vi "configureTriggering.vi"(8 "error in (no error)":errorcluster, 10 "channel":i32, 11 "K2602 in":refnum<class "K2602.lvclass">) -> (0 "error out":errorcluster, 3 "K2602 out":refnum<class "K2602.lvclass">)   [LabVIEW 2009, in "Hardware.lvlib" / "Channels.lvlib" / "K2602.lvclass"]
uses:
  K2602.lvclass
  K2602.lvclass/K2602.ctl
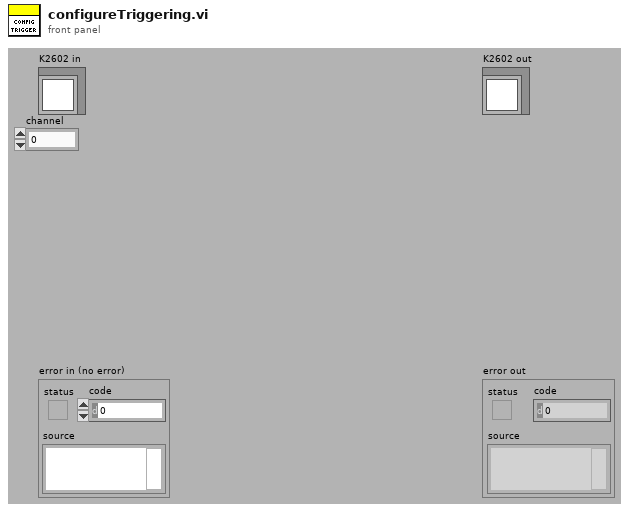
[diagram p1: front panel]
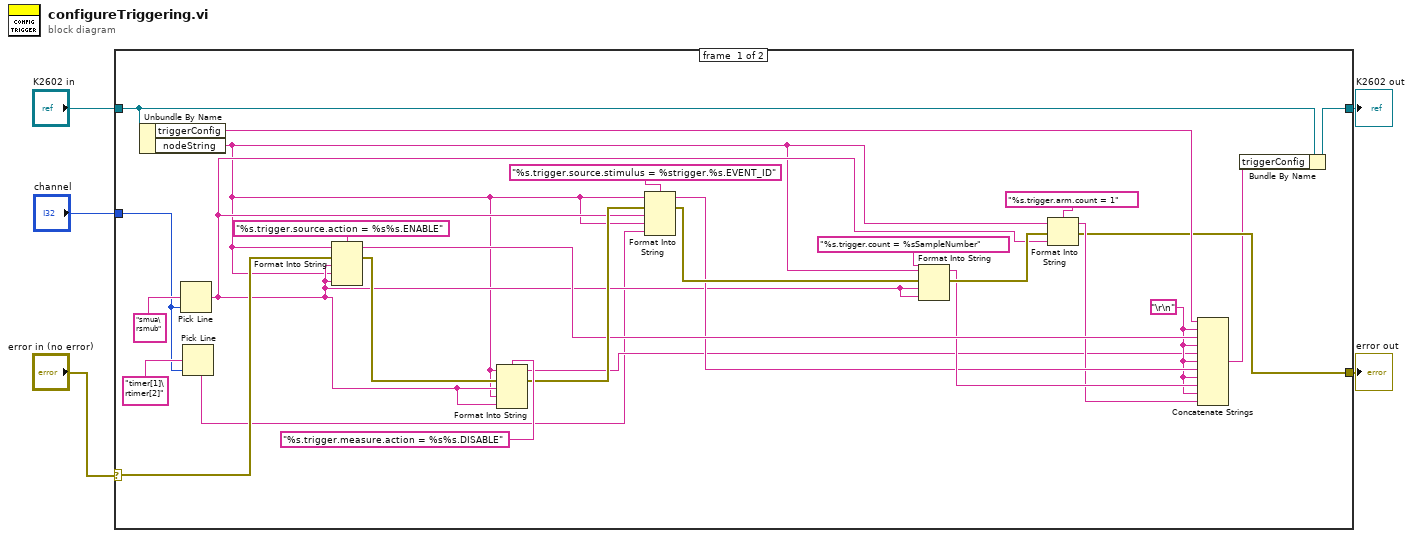
[diagram p0: block diagram]
diagram:
  n1 = case shown="No Error" "error in (no error)" {
    selector: "error in (no error)" -> [w30 w34]
    tunnel: [w14 w34] -> w4
    tunnel: [w11 w33] -> w2
    tunnel: "K2602 in" -> [w12 w33]
    tunnel: "channel" -> [w24 _]
    frame #0 {
      w10 = "\r\n"
      n2 = Unbundle By Name(w12) -> ("triggerConfig"=w19:string, "nodeString"=w6:string)
      n3 = Pick Line(multi-line string="smua\rsmub" ("options"), line index=w24) -> (output string=w8:string)  [unwired: 1 out]
      n4 = Pick Line(multi-line string="timer[1]\rtimer[2]" ("options"), line index=w24) -> (output string=w7:string)  [unwired: 1 out]
      n5 = Format Into String(format string="%s.trigger.source.action = %s%s.ENABLE", initial string=w6, error in=w30, w8, w6, w8) -> (resulting string=w18:string, error out=w28:errorcluster)
      n6 = Format Into String(format string="%s.trigger.measure.action = %s%s.DISABLE", initial string=w6, error in=w28, w8, w6, w8) -> (resulting string=w9:string, error out=w26:errorcluster)
      n7 = Format Into String(format string="%s.trigger.source.stimulus = %strigger.%s.EVENT_ID", initial string=w6, error in=w26, w8, w6, w7) -> (resulting string=w16:string, error out=w20:errorcluster)
      n8 = Format Into String(format string="%s.trigger.count = %sSampleNumber", initial string=w6, error in=w20, w8, w8) -> (resulting string=w17:string, error out=w21:errorcluster)
      n9 = Format Into String(format string="%s.trigger.arm.count = 1", initial string=w6, error in=w21, w8) -> (resulting string=w15:string, error out=w14:errorcluster)
      n10 = Concatenate Strings(w19, w10, w18, w10, w9, w10, w16, w10, w17, w10, w15) -> (w13:string)
      n11 = Bundle By Name(cluster=w12, "triggerConfig"=w13) -> (w11:refnum<class "K2602.lvclass">)
    }
    frame #1 {
    }
  }
  "error out" <- w4
  "K2602 out" <- w2
